vi "FindWorkingZDistance.vi"(5 "Template File Path":path=path "C:/Users/Aerotech/Documents/BNL_ThermomechanicalStave/0_Calibration/1_Camera", 8 "error in":errorcluster, 9 "Circle Fit Options":T10={"Process"=enum."Get Best Edge", "Step Size"=3.0, "Max Pixel Radius"=3}, 11 "Images Directory":path=path "C:/Users/Aerotech/Documents/Stave Assembly Records/2017-03-06/autofocusing") -> (0 "error out":errorcluster, 1 "Radius vs Height: Linear Fit Results":T15, 2 "Uncertainty on optimized Z":dbl, 3 "Optimized Z":dbl)   [LabVIEW 2016]
uses:
  <vilib>/vision/Image Controls.llb/IMAQ Image.ctl
  <vilib>/vision/Measure.llb/Edge Options.ctl
  <vilib>/vision/Measure.llb/Edge Polarity.ctl
  <vilib>/Utility/file.llb/Read Delimited Spreadsheet (DBL).vi
  <vilib>/regexp/Match Regular Expression.xnode
  <vilib>/Analysis/NI_AALPro.lvlib
panel:
  in  "Tab Control: Plots":T1(tab)
  out "Normalized Intensity vs Radius":T2(graph)
  out "Derivative: Normalized Intensity vs Radius":T3(graph)
  out "Fitted SD dI/dR vs Z":T3(graph)
  out "Location of minimum":dbl
  out "Uncertainty on minimum location":dbl
  out "Fitted radii vs Z":T3(graph)
  in  "Tab Control":T4(tab)
  out "Capture coordinates":dbl[][](array[numeric])
  out "Search running?":bool
  out "Finished!":bool
  out "Processing Image #":i32
  out "Search image out":T5(plugin-control)
  in  "Circle Finding Options":T8={"Search  Direction"=1, "Edge Options"={"Edge Polarity"=2, "Kernel Size"=3, "Width"=3, "Minimum Edge Strength"=10.0, "Interpolation Type"=enum."Bilinear Fixed", "Data Processing Method"=enum."Average"}, "Show Search Area"=FALSE, "Show Search Lines"=FALSE, "Show Edges Found"=FALSE, "Show Result"=TRUE, "Search Area Color"=65280, "Search Lines Color"=255, "Edge Locations Color"=16776960, "Result Color"=65511, "Overlay Group Name"=""} {"Search  Direction" items=["Outside to Inside", "Inside to Outside"]; "Edge Options"."Edge Polarity" items=["All Edges", "Rising Edges", "Falling Edges"]; "Edge Options"."Minimum Edge Strength" format="%.2f"; "Edge Options"."Width" step=2; "Edge Options"."Kernel Size" step=2}
  in  "Circle ROI Descriptor":T9={"Global Rectangle"=[675, 567, 1751, 1642], "Contours"=[{"ID"=enum."External", "Type"=7, "Coordinates"=[1212, 1104, 85, 537, 0, 0]}]} {"Contours"."Type" items=["No Selection", "Point", "Line", "Rectangle", "Oval", "Polygon", "Freehand Region", "Annulus", "Unused2", "Unused3", "Broken Line", "Freehand Line", "Rotated Rectangle"]}
  in  "Pattern Match Settings":T11={"Algorithm"=2, "Number of Matches Requested"=1, "Minimum Match Score"=700.0, "SubPixel Accuracy"=TRUE, "Rotation Angle Ranges"=[{"Start"=0.0, "End"=360.0}], "Show Search Area"=FALSE, "Show Result"=TRUE} {"Rotation Angle Ranges"."End" format="%.1f"; "Rotation Angle Ranges"."Start" format="%.1f"; "Minimum Match Score" min=0 max=1000 format="%.2f"; "Number of Matches Requested" min=1; "Algorithm" items=["All", "Low Discrepancy Sampling", "Grayscale Value Pyramid", "Gradients Pyramid"]}
  in  "Intensity vs Radius Binning":T12={"nBins"=440.0, "Min radius [pixels]"=0.0, "Max radius [pixels]"=440.0}
  out "Fitted Circle":T13 {"Average SNR (dB)" format="%.2f"; "Average Strength" format="%.2f"; "Roundness (Real-World)" format="%.2f"; "Radius (Real-World)" format="%.2f"; "Center (Real-World)"."Y" format="%.2f"; "Center (Real-World)"."X" format="%.2f"; "Radius (Pixels)" format="%.2f"; "Center (Pixels)"."Y" format="%.2f"; "Center (Pixels)"."X" format="%.2f"}
  in  "Naming Convention":string="*.png"
  in  "Minimization inputs":T14={"Minimizing alg"=0, "Search start"=0.0, "Search end"=1.0, "Search accuracy"=1e-08, "Step type"=0} {"Step type" items=["fixed function", "modified function"]; "Search accuracy" format="%.2e"; "Search end" format="%.2f"; "Search start" format="%.2f"; "Minimizing alg" items=["Golden Section Search", "Brent with Derivatives"]}
  out "delta Fitted SD( -dI/dR )":dbl[](array[numeric])
  out "delta Fitted edge locations [pixels]":dbl[](array[numeric])
  out "Fitted SD( -dI/dR )":dbl[](array[numeric])
  out "Fitted edge locations [pixels]":dbl[](array[numeric])
  out "Template Image":T5
  # "FIND CAMERA WORKING DISTANCE Brandeis University - Brookhaven National Laboratory * ATLAS Phase II Inner Tracker Upgrade"
  # "Inner 85\nOuter 537"
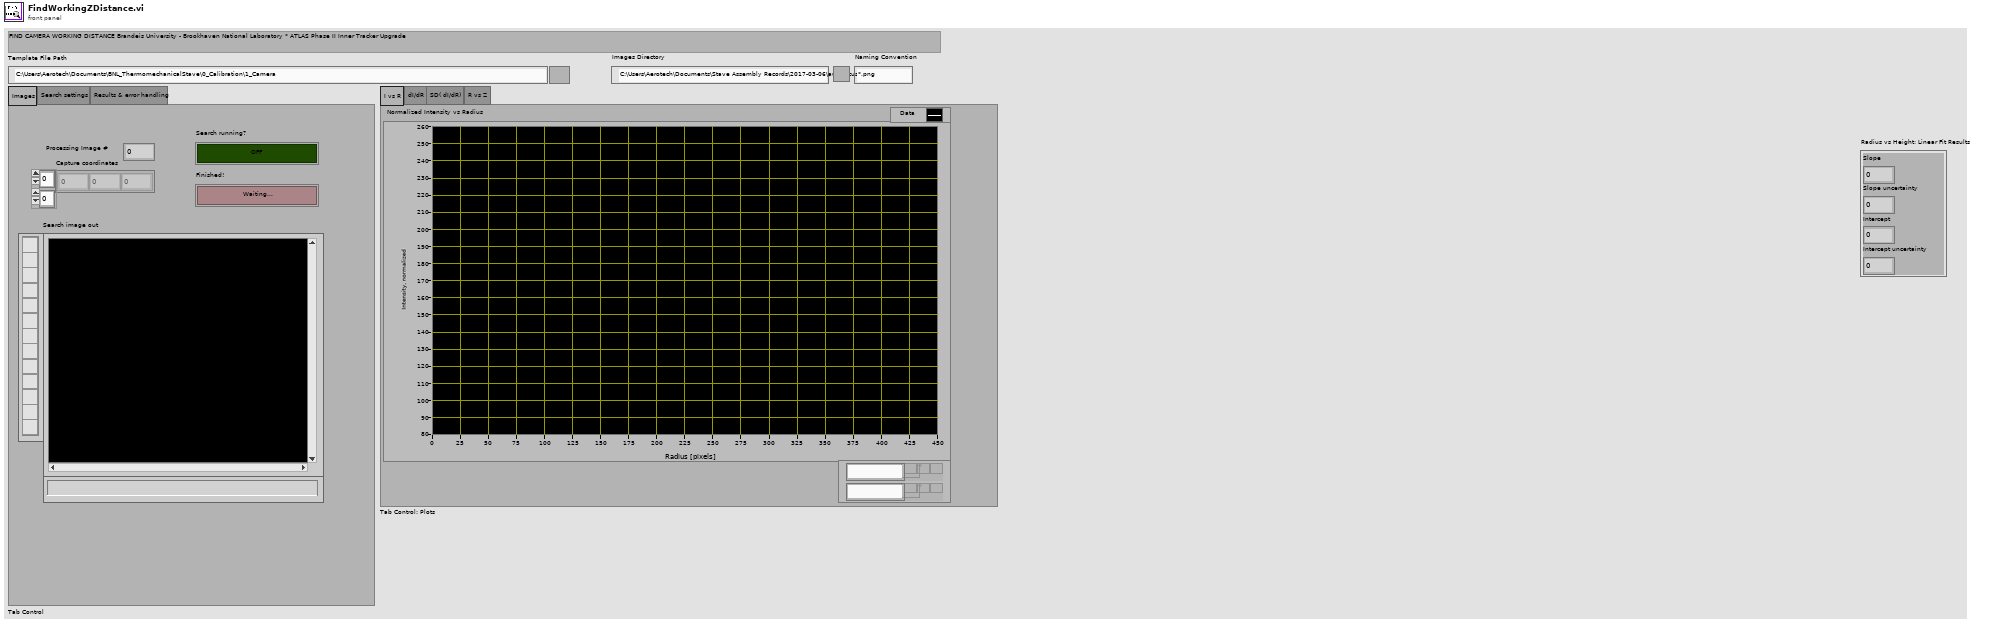
[diagram p1: front panel]
types:
  T1 = enum32{"I vs R", "dI/dR", "SD( dI/dR)", "R vs Z"}
  T2 = cluster{"Radius bins":dbl[], "Normalized Intensity":dbl[]}
  T3 = cluster{"Radius bins":dbl[], "Best Gaussian Fit":dbl[]}[]
  T4 = enum32{"Images", "Search settings", "Results & error handling"}
  T5 = typedef "IMAQ Image.ctl" = refnum<image>
  T6 = typedef "Edge Options.ctl" = cluster{"Edge Polarity":T7, "Kernel Size":u32, "Width":u32, "Minimum Edge Strength":sgl, "Interpolation Type":enum32{"Zero Order", "Bilinear", "Quadratic", "Cubic", "Bilinear Fixed"}, "Data Processing Method":enum32{"Average", "Median"}}
  T7 = typedef "Edge Polarity.ctl" = u32
  T8 = cluster{"Search  Direction":u32, "Edge Options":T6, "Show Search Area":bool, "Show Search Lines":bool, "Show Edges Found":bool, "Show Result":bool, "Search Area Color":u32, "Search Lines Color":u32, "Edge Locations Color":u32, "Result Color":u32, "Overlay Group Name":string}
  T9 = cluster{"Global Rectangle":i32[], "Contours":cluster{"ID":enum32{"External", "Internal"}, "Type":u32, "Coordinates":i32[]}[]}
  T10 = cluster{"Process":enum16{"Get First Edge", "Get First + Last Edge", "Get All Edges", "Get Best Edge"}, "Step Size":dbl, "Max Pixel Radius":i32}
  T11 = cluster{"Algorithm":i32, "Number of Matches Requested":i32, "Minimum Match Score":sgl, "SubPixel Accuracy":bool, "Rotation Angle Ranges":cluster{"Start":sgl, "End":sgl}[], "Show Search Area":bool, "Show Result":bool}
  T12 = cluster{"nBins":dbl, "Min radius [pixels]":dbl, "Max radius [pixels]":dbl}
  T13 = cluster{"Center (Pixels)":cluster{"X":sgl, "Y":sgl}, "Radius (Pixels)":dbl, "Center (Real-World)":cluster{"X":sgl, "Y":sgl}, "Radius (Real-World)":dbl, "Roundness (Real-World)":dbl, "Average Strength":dbl, "Average SNR (dB)":dbl}
  T14 = cluster{"Minimizing alg":u16, "Search start":dbl, "Search end":dbl, "Search accuracy":dbl, "Step type":u16}
  T15 = cluster{"Slope":dbl, "Slope uncertainty":dbl, "Intercept":dbl, "Intercept uncertainty":dbl}
  T16 = cluster{"initial amplitude":dbl, "initial center":dbl, "initial standard deviation":dbl, "offset":dbl}
  T17 = cluster{"slope":dbl, "delta slope":dbl, "intercept":dbl, "delta intercept":dbl}
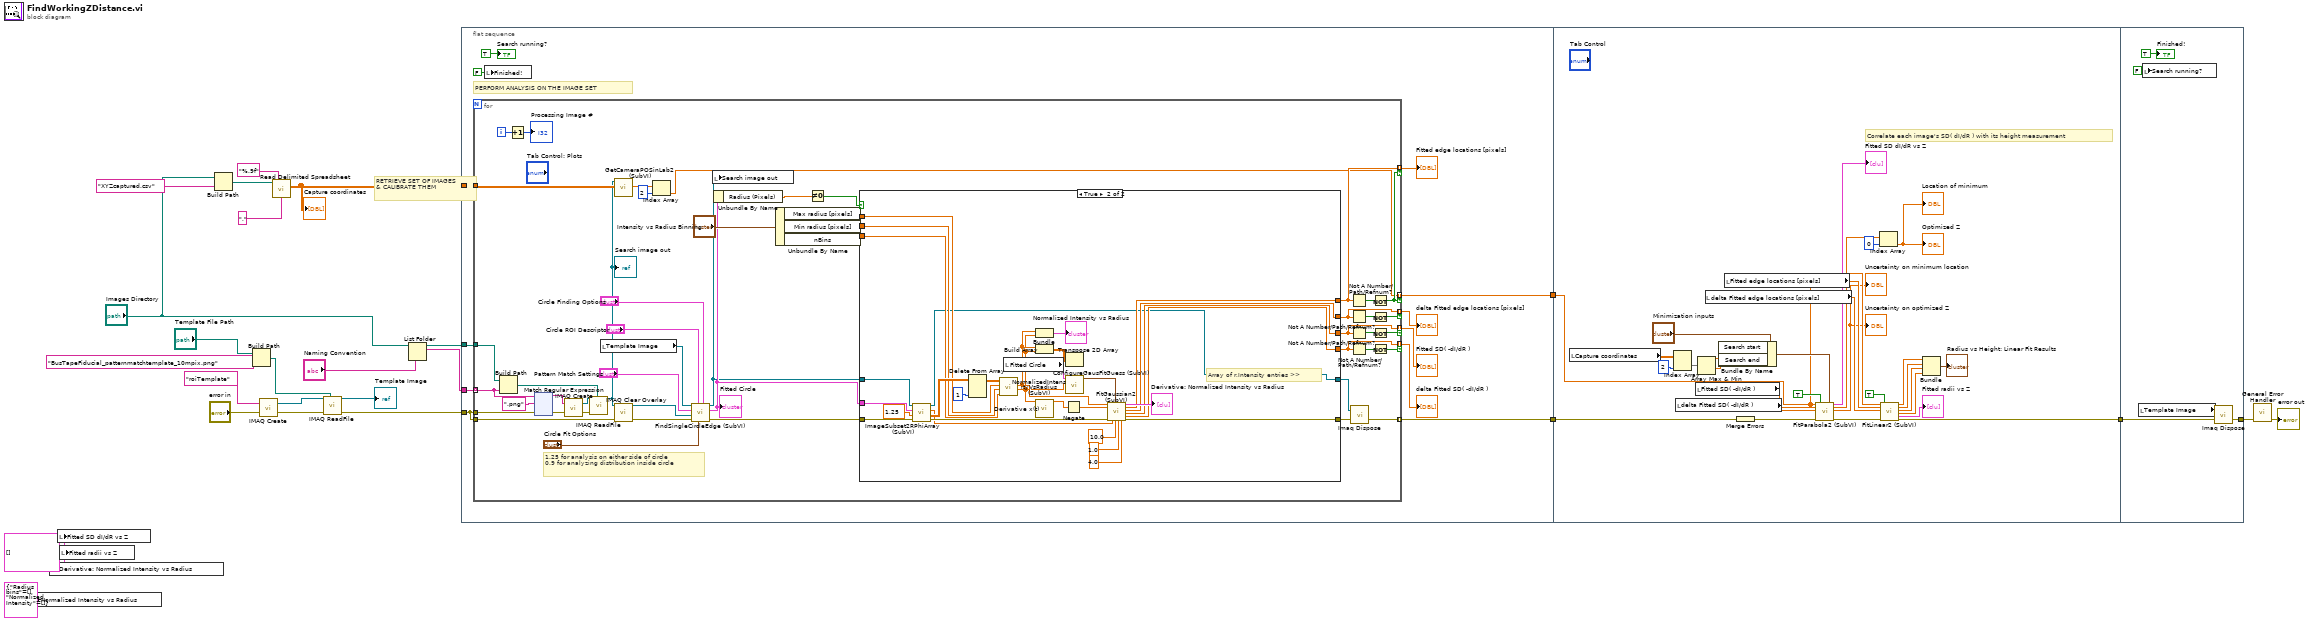
[diagram p0: block diagram]
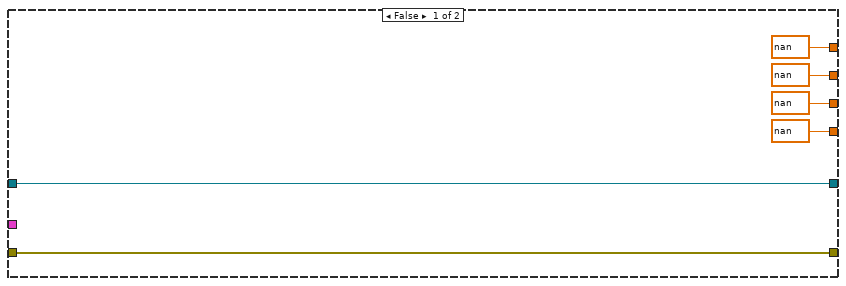
[diagram p2: hidden frame]
diagram:
  w12 = T3 [] ("Fitted SD dI/dR vs Z")
  # "RETRIEVE SET OF IMAGES\n& CALIBRATE THEM"
  n1 = local write "Normalized Intensity vs Radius"(T2 {"Radius bins"=[], "Normalized Intensity"=[]} ("Normalized Intensity vs Radius")) -> ()
  n2 = local write "Derivative: Normalized Intensity vs Radius"(w12) -> ()
  n3 = local write "Fitted SD dI/dR vs Z"(w12) -> ()
  n4 = local write "Fitted radii vs Z"(w12) -> ()
  n5 = Build Path(base path="Images Directory", name or relative path="XYZcaptured.csv") -> (appended path=w10:path)
  n6 = Build Path(base path="Template File Path", name or relative path="BusTapeFiducial_patternmatchtemplate_10mpix.png") -> (appended path=w16:path)
  n7 = call "IMAQ Create"("Image Name"="roiTemplate", "error in (no error)"="error in") -> ("New Image"=w22:T5, "error out"=w23:errorcluster)  [unwired: 3 in]
  n8 = call-poly <vilib>:"Read Delimited Spreadsheet.vi"("file path (dialog if empty)"=w10, "format (%.3f)"="%.9f", "delimiter (\\t)"="," ("delimiter (\\t)")) -> ("all rows"=w2:dbl[][])  [unwired: 7 in, 5 out]
  "Capture coordinates" <- w2
  n9 = call "IMAQ ReadFile"("File Path"=w16, "error in (no error)"=w23, "Image"=w22) -> ("error out"=w15:errorcluster, "Image Out"=→"Template Image":T5)  [unwired: 4 in, 3 out]
  n10 = List Folder(path="Images Directory", pattern="Naming Convention") -> (path out=w4:path, filenames=w3:string[])  [unwired: 2 in, 2 out]
  n11 = flat-sequence {
    tunnel: w15 -> [w27]
    tunnel: w2 -> [w35]
    tunnel: [w34] -> w19
    tunnel: [w29] -> w13
    tunnel: w3 -> [w28]
    tunnel: w4 -> [w26]
    tunnel: [w252] -> w20
    tunnel: w19 -> [w264]
    tunnel: w13 -> [w239]
    tunnel: [w265] -> w1
    tunnel: w20 -> [w266]
    frame #0 {
      # "PERFORM ANALYSIS ON THE IMAGE SET"
      n12 = for {
        tunnel: w27 -> [w72]
        tunnel: w35 -> [w78]
        tunnel: [w54] -> w34 mode=indexing
        tunnel: [w58] -> w33 mode=indexing if=w57
        tunnel: [w59] -> w32 mode=indexing if=w63
        tunnel: [w61] -> w31 mode=indexing if=w60
        tunnel: [w66] -> w30 mode=indexing if=w53
        tunnel: [w52] -> w29 mode=indexing if=w53
        tunnel: w28 -> [w42] mode=indexing
        tunnel: w27 -> [w41]
        tunnel: w26 -> [w40]
        i -> [w39]
        # "1.25 for analysis on either side of circle\n0.9 for analyzing distribution inside circle"
        n13 = Build Path(base path=w40, name or relative path=w42) -> (appended path=w47:path)
        n14 = Increment(x=w39) -> (x+1=→"Processing Image #":i32)
        n15 = xnode "Match Regular Expression"("input string"=w42, "regular expression"=".png", "error in"=w41) -> ("before match"=w45:string, "error out"=w44:errorcluster)  [unwired: 3 in, 3 out]
        n16 = call "IMAQ Create"("Image Name"=w45, "error in (no error)"=w44) -> ("New Image"=w48:T5, "error out"=w49:errorcluster)  [unwired: 3 in]
        n17 = call "IMAQ ReadFile"("File Path"=w47, "error in (no error)"=w49, "Image"=w48) -> ("Image Out"=w43:T5)  [unwired: 4 in, 4 out]
        "Search image out" <- w43
        n18 = local read "Template Image"() -> (w85:T5)
        n19 = call "GetCameraPOSinLab2 (SubVI).vi"("Loaded array"=w78, "Refnum in"=w43) -> ("Image coordinates in lab frame"=w79:dbl[])  [unwired: 7 in, 2 out]
        n20 = call "IMAQ Clear Overlay"("error in (no error)"=w72, "Image"=w43) -> ("error out"=w71:errorcluster, "Image Out"=w73:T5)  [unwired: 8 in]
        n21 = Index Array(array=w79, index=2 ("disabled index (col)")) -> (element=w52:dbl)
        n22 = call "FindSingleCircleEdge (SubVI).vi"("Circle Finding Options"="Circle Finding Options", "Circle Fit Options"="Circle Fit Options", "Circle ROI Descriptor"="Circle ROI Descriptor", "error in (no error)"=w71, "Search Image in"=w73, "Pattern Match Settings"="Pattern Match Settings", "Template in"=w85) -> ("error out"=w80:errorcluster, "Fitted Circle"=w70:T13, "Search image out"=w50:T5)  [unwired: 2 in]
        "Fitted Circle" <- w70
        n23 = local write "Search image out"(w50) -> ()
        n24 = Unbundle By Name(w70) -> ("Radius (Pixels)"=w69:dbl)
        n25 = Unbundle By Name("Intensity vs Radius Binning") -> ("Max radius [pixels]"=w75:dbl, "Min radius [pixels]"=w74:dbl, "nBins"=w76:dbl)
        n26 = Not Equal To 0?(x=w69) -> (x != 0?=w68:bool)
        n27 = case shown="True" w68 {
          tunnel: w80 -> [w200 w235]
          tunnel: w50 -> [w201 w234]
          tunnel: [nan ("delta center") w224] -> w58
          tunnel: [nan ("standard deviation") w223] -> w59
          tunnel: [nan ("delta standard deviation") w222] -> w61
          tunnel: w76 -> [_ w216]
          tunnel: w75 -> [_ w215]
          tunnel: w74 -> [_ w214]
          tunnel: [nan ("center") w213] -> w66
          tunnel: w70 -> [_ w209]
          tunnel: [w201 w207] -> w56
          tunnel: [w200 w206] -> w55
          frame False {
          }
          frame True {
            # "Array of r,Intensity entries >>"
            n28 = call "ImageSubset2RPhiArray (SubVI).vi"("error in (no error)"=w235, "Multiplier for Radius"=1.25, "Fitted Circle"=w209, "Full Image in"=w234) -> ("error out"=w221:errorcluster, "2D Array: r, phi, intensity"=w225:dbl[][], "Radius (Pixels)"=w217:dbl, "Subset image out"=w207:T5)  [unwired: 4 in]
            n29 = Delete From Array(array=w225, index (col)=1 ("disabled index (col)")) -> (array with subset deleted=w228:dbl[][])  [unwired: 2 in, 1 out]
            n30 = call "NormalizedIntensityVsRadius (SubVI).vi"("nBins"=w216, "Min"=w214, "Max"=w215, "Input Array (r,I)"=w228) -> ("Normalized Intensity"=w210:dbl[], "Radius bins"=w211:dbl[])  [unwired: 5 in, 1 out]
            n31 = local read "Fitted Circle"() -> (w229:T13)
            n32 = Bundle("Radius bins"=w211, "Normalized Intensity"=w210) -> (→"Normalized Intensity vs Radius":T2)  [unwired: 1 in]
            n33 = Build Array(w211, w210) -> (w227:dbl[][])
            n34 = call <vilib>:"Derivative x(t).vi"("X"=w210) -> ("dX/dt"=w232:dbl[])  [unwired: 9 in, 1 out]
            n35 = Negate(x=w232) -> (-x=w226:dbl[])
            n36 = Transpose 2D Array(2D array=w227) -> ()  [unwired: 1 out]
            n37 = call "ConfigureGausFitGuess (SubVI).vi"("Array"=w210, "Fitted Circle"=w229) -> ("initial guess out"=w230:T16)  [unwired: 9 in]
            n38 = call "FitGaussian2 (SubVI).vi"("x values"=w211, "y values"=w226, "error in"=w221, "Estimated mean"=w217, "initial guess"=w230, "Estimated width"=10.0, "Nsigma Low"=1.0, "Nsigma High"=4.0) -> ("Plot with Gaussian fit"=→"Derivative: Normalized Intensity vs Radius":T3, "center"=w213:dbl, "delta center"=w224:dbl, "standard deviation"=w223:dbl, "delta standard deviation"=w222:dbl, "error out"=w206:errorcluster)  [unwired: 6 in]
          }
        }
        n39 = Not A Number/Path/Refnum?(number/path/refnum=w66) -> (NaN/Path/Refnum?=w67:bool)
        n40 = Not A Number/Path/Refnum?(number/path/refnum=w58) -> (NaN/Path/Refnum?=w65:bool)
        n41 = Not A Number/Path/Refnum?(number/path/refnum=w59) -> (NaN/Path/Refnum?=w64:bool)
        n42 = Not A Number/Path/Refnum?(number/path/refnum=w61) -> (NaN/Path/Refnum?=w62:bool)
        n43 = call "Imaq Dispose"("Image"=w56, "error in (no error)"=w55) -> ("error out"=w54:errorcluster)  [unwired: 4 in]
        n44 = Not(x=w67) -> (.not. x?=w53:bool)
        n45 = Not(x=w65) -> (.not. x?=w57:bool)
        n46 = Not(x=w64) -> (.not. x?=w63:bool)
        n47 = Not(x=w62) -> (.not. x?=w60:bool)
      }
      "Fitted edge locations [pixels]" <- w30
      "Fitted SD( -dI/dR )" <- w32
      "delta Fitted edge locations [pixels]" <- w33
      "delta Fitted SD( -dI/dR )" <- w31
      n48 = local write "Finished!"(FALSE ("Review")) -> ()
      "Search running?" <- TRUE ("Search running?")
    }
    frame #1 {
      # "Correlate each image's SD( dI/dR ) with its height measurement"
      n49 = local read "Capture coordinates"() -> (w246:dbl[][])
      n50 = Index Array(array=w246, index (col)=2 ("disabled index (col)")) -> (element=w244:dbl[])  [unwired: 1 in]
      n51 = local read "delta Fitted SD( -dI/dR )"() -> (w258:dbl[])
      n52 = local read "Fitted SD( -dI/dR )"() -> (w259:dbl[])
      n53 = Array Max & Min(array=w244) -> (max value=w242:dbl, min value=w243:dbl)  [unwired: 2 out]
      n54 = local read "delta Fitted edge locations [pixels]"() -> (w256:dbl[])
      n55 = Bundle By Name(cluster="Minimization inputs", "Search start"=w243, "Search end"=w242) -> (w240:T14)
      n56 = local read "Fitted edge locations [pixels]"() -> (w257:dbl[])
      n57 = Merge Errors(w264) -> (w260:errorcluster)
      n58 = call "FitParabola2 (SubVI).vi"("x values"=w239, "y values"=w259, "delta y values"=w258, "error in"=w260, "Use all points"=TRUE, "Minimization inputs"=w240) -> ("Plot with quadratic fit"=→"Fitted SD dI/dR vs Z":T3, "Minima"=w262:dbl[], "Uncertainty on minimum"=→"Uncertainty on optimized Z" →"Uncertainty on minimum location":dbl, "error out"=w253:errorcluster)  [unwired: 10 in]
      n59 = Index Array(array=w262, index=0) -> (element=→"Optimized Z" →"Location of minimum":dbl)
      n60 = call "FitLinear2 (SubVI).vi"("x values"=w239, "y values"=w257, "delta y values"=w256, "error in"=w253, "Use all points"=TRUE) -> ("slope"=w251:dbl, "delta slope"=w250:dbl, "intercept"=w249:dbl, "delta intercept"=w248:dbl, "Plot with linear fit"=→"Fitted radii vs Z":T3, "error out"=w252:errorcluster)  [unwired: 9 in]
      n61 = Bundle("slope"=w251, "delta slope"=w250, "intercept"=w249, "delta intercept"=w248) -> (→"Radius vs Height: Linear Fit Results":T17)  [unwired: 1 in]
    }
    frame #2 {
      n62 = local read "Template Image"() -> (w267:T5)
      n63 = local write "Search running?"(FALSE ("Search running?")) -> ()
      n64 = call "Imaq Dispose"("Image"=w267, "error in (no error)"=w266) -> ("error out"=w265:errorcluster)  [unwired: 4 in]
      "Finished!" <- TRUE ("Review")
    }
  }
  n65 = call <vilib>:"General Error Handler.vi"("error in (no error)"=w1) -> ("error out"=→"error out":errorcluster)  [unwired: 10 in, 4 out]
